vi "Build Text.vi"(0 "Beginning Text":string, 5 "sdhg":string, 11 "error in (no error)":errorcluster) -> (4 "Result":string, 15 "error out":errorcluster)   [LabVIEW 2023]
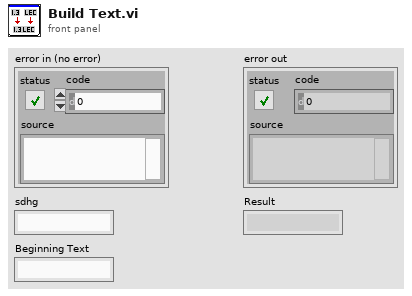
[diagram p1: front panel]
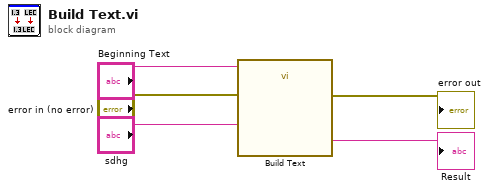
[diagram p0: block diagram]
diagram:
  n1 = call "Build Text"("Beginning Text"="Beginning Text", "sdhg"="sdhg", "error in (no error)"="error in (no error)") -> ("Result"=→"Result":string, "error out"=→"error out":errorcluster)  [unwired: 11 in]
